vi "set_zoom.vi"(8 "error in (no error)":errorcluster, 10 "zoom":dbl, 11 "FPGAWrapperMH120124FrameScan_PXI7813R in":refnum<class "FPGAWrapperMH120124FrameScan_PXI7813R.lvclass">) -> (0 "error out":errorcluster, 3 "FPGAWrapperMH120124FrameScan_PXI7813R out":refnum<class "FPGAWrapperMH120124FrameScan_PXI7813R.lvclass">)   [LabVIEW 2010, in "FPGAWrapperMH120124FrameScan_PXI7813R.lvclass"]
uses:
  FPGAWrapperMH120124FrameScan_PXI7813R.lvclass
  FPGAWrapperMH120124FrameScan_PXI7813R.lvclass/FPGAWrapperMH120124FrameScan_PXI7813R.ctl
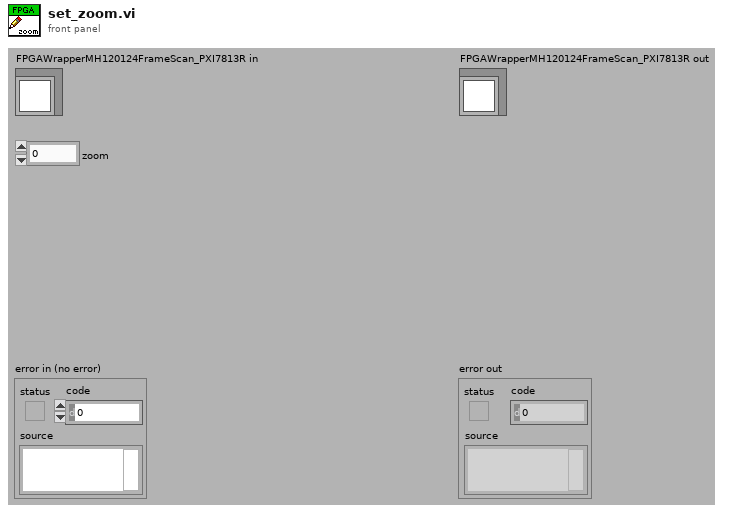
[diagram p1: front panel]
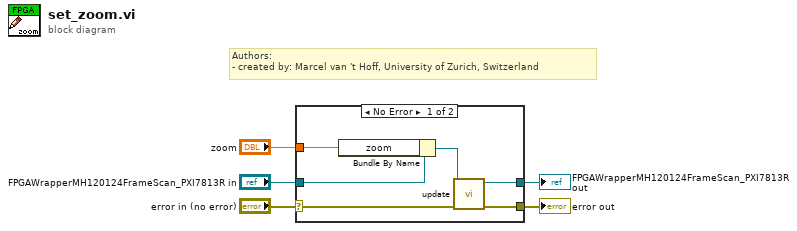
[diagram p0: block diagram]
diagram:
  # "Authors: \n- created by: Marcel van 't Hoff, University of Zurich, Switzerland"
  n1 = case shown="No Error" "error in (no error)" {
    selector: "error in (no error)" -> [w7 w12]
    tunnel: [w6 w12] -> w4
    tunnel: [w8 w13] -> w2
    tunnel: "FPGAWrapperMH120124FrameScan_PXI7813R in" -> [w11 w13]
    tunnel: "zoom" -> [w10 _]
    frame No Error {
      n2 = Bundle By Name(cluster=w11, "zoom"=w10) -> (w9:refnum<class "FPGAWrapperMH120124FrameScan_PXI7813R.lvclass">)
      n3 = call-dynamic "update.vi"("error in (no error)"=w7, "FPGAWrapperMH120124FrameScan_PXI7813R in"=w9) -> ("error out"=w6:errorcluster, "FPGAWrapperMH120124FrameScan_PXI7813R out"=w8:refnum<class "FPGAWrapperMH120124FrameScan_PXI7813R.lvclass">)  [unwired: 8 in]
    }
    frame Error {
    }
  }
  "error out" <- w4
  "FPGAWrapperMH120124FrameScan_PXI7813R out" <- w2
